vi "FPGA Toplevel.vi"() -> ()   [LabVIEW 2012]
uses:
  <vilib>/LabVIEW Targets/FPGA/RIO/BlueMoonOnboardIO/nicrio_cRIO-BlueMoonOnboardAi_TerminalMod.ctl
  <vilib>/LabVIEW Targets/FPGA/RIO/BlueMoonOnboardIO/nicrio_cRIO-BlueMoonOnboardAi_VoltageRange.ctl
  <vilib>/IEDriver/SPIandI2C/FPGA/Private/Initialize Port (I2C).vi
  <vilib>/IEDriver/SPIandI2C/FPGA/Private/IP Port (I2C).vi
  <vilib>/IEDriver/SPIandI2C/FPGA/Private/Configure Port (I2C).vi
  <vilib>/IEDriver/SPIandI2C/FPGA/Private/Read Port (I2C).vi
  <vilib>/IEDriver/SPIandI2C/FPGA/Private/Arm Port (I2C).vi
  <vilib>/IEDriver/SPIandI2C/FPGA/Private/Write Port (I2C).vi
  <vilib>/rvi/Emulation/niFpgaSctlEmulationGetInTimedLoop.vi
  <vilib>/rvi/Emulation/niFpgaSctlEmulationGlobalWrite.vi
  <vilib>/robotics/Utilities/FPGA Utilities/Generate Digital Pulse (uSec).vi
  <vilib>/rvi/eio/common/nirviEmuTemplateMethod_errors.vi
  <vilib>/rvi/eio/common/nirviEmuTemplatePropertySet_noerrors.vi
  <vilib>/eio/EIONode/EIONode.xnode
  <vilib>/eio/EIOPropertyNode/EIOPropertyNode.xnode
  <vilib>/rvi/eio/common/nirviEmuTemplatePropertyGet_errors.vi
  <vilib>/rvi/eio/common/nirviEmuTemplatePropertyGet_noerrors.vi
  <vilib>/rvi/eio/common/nirviEmuTemplatePropertySet_errors.vi
  <vilib>/robotics/Utilities/FPGA Utilities/NI_Robotics_FPGA Utilities.lvlib
  <vilib>/IEDriver/SPIandI2C/FPGA/Library/IP SPI&I2C.lvlib
panel:
  in  "servo Claw":u32=1500
  in  "Count(uSec) Claw":u32=5000
  in  "servo Arm":u32=1500
  in  "Count(uSec) Arm":u32=5000
  in  "Sensor time(us)":u16=1000 caption="Count(uSec)"
  in  "Calibration Parameters":T1={"m"=3.028200149536133, "b"=0.30049991607666016, "k"=0.04309988021850586}
  in  "Write Address":u8
  in  "Write Data In":u8
  out "Read Data out":u8
  in  "Read Address":u8
  in  "Mouse Action":T2(ring)
  out "IR 5":fxp<+/-,24,5>
  out "IR 4":fxp<+/-,24,5>
  out "IR 3":fxp<+/-,24,5>
  out "IR 2":fxp<+/-,24,5>
  in  "I2C Protocol Action 0":T3(ring)=enum."Idle"
  in  "I2C Protocol Input Data 0":u8
  out "I2C Protocol Output Data 0":u8
  in  "I2C Protocol Configure 0":T4 {"Command (Write & Read)" items=["Write & Read", "Write", "Read"]}
  out "IR 1":fxp<+/-,24,5>
  in  "Motor 4":T5={"Period (us)"=5000, "Pulse width (us)"=2502}
  in  "Motor 3":T5={"Period (us)"=5000, "Pulse width (us)"=2502}
  in  "Motor 2":T5={"Period (us)"=5000, "Pulse width (us)"=2502}
  in  "Enable":bool
  in  "Motor 1":refnum<k21>="DIO5"
  in  "Motor 1":T5={"Period (us)"=5000, "Pulse width (us)"=2502}
  in  "Enable":refnum<k21>="DIO4"
  in  "Motor 4":refnum<k21>="DIO8"
  in  "Motor 3":refnum<k21>="DIO7"
  in  "Motor 2":refnum<k21>="DIO6"
  out "IR 0":fxp<+/-,24,5>
  # "Mouse"
  # "Servo"
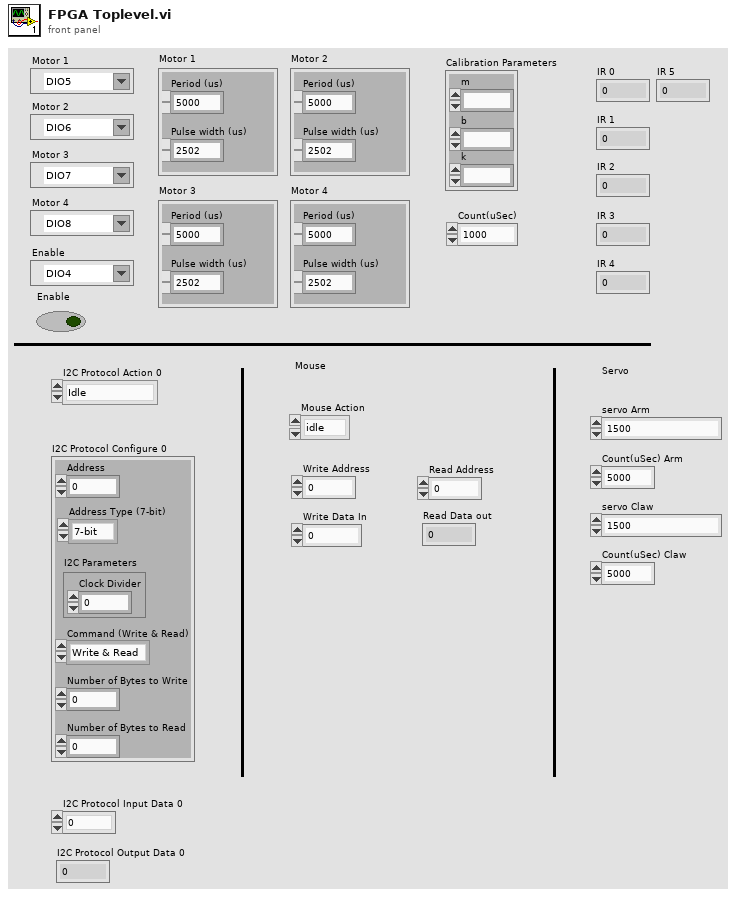
[diagram p1: front panel]
types:
  T1 = cluster{"m":fxp<+/-,26,5>, "b":fxp<+/-,26,5>, "k":fxp<+/-,26,5>}
  T2 = enum16{"idle", "set idle", "begin", "write", "read", "power down", "reset"}
  T3 = enum8{"Configure", "Write", "Arm", "Read", "Set Idle", "Idle"}
  T4 = cluster{"Address":u16, "Address Type (7-bit)":enum16{"7-bit", "10-bit"}, "I2C Parameters":cluster{"Clock Divider":u32}, "Command (Write & Read)":u8, "Number of Bytes to Write":u16, "Number of Bytes to Read":u16}
  T5 = cluster{"Period (us)":u32, "Pulse width (us)":u32}
  T6 = cluster{"SCL":refnum<k21>, "SDA":refnum<k21>, "PD":refnum<k21>}
  T7 = typedef "nicrio_cRIO-BlueMoonOnboardAi_TerminalMod.ctl" = u8
  T8 = typedef "nicrio_cRIO-BlueMoonOnboardAi_VoltageRange.ctl" = u8
  T9 = typedef "IP SPI&I2C.lvlib/Private Data (I2C).ctl" = cluster{"Arm Trigger":refnum<k21>, "API to IP Data":refnum<k21>, "IP to API Data":refnum<k21>, "Configuration Register":refnum<k21>, "Configuration Lock":refnum<k21>}
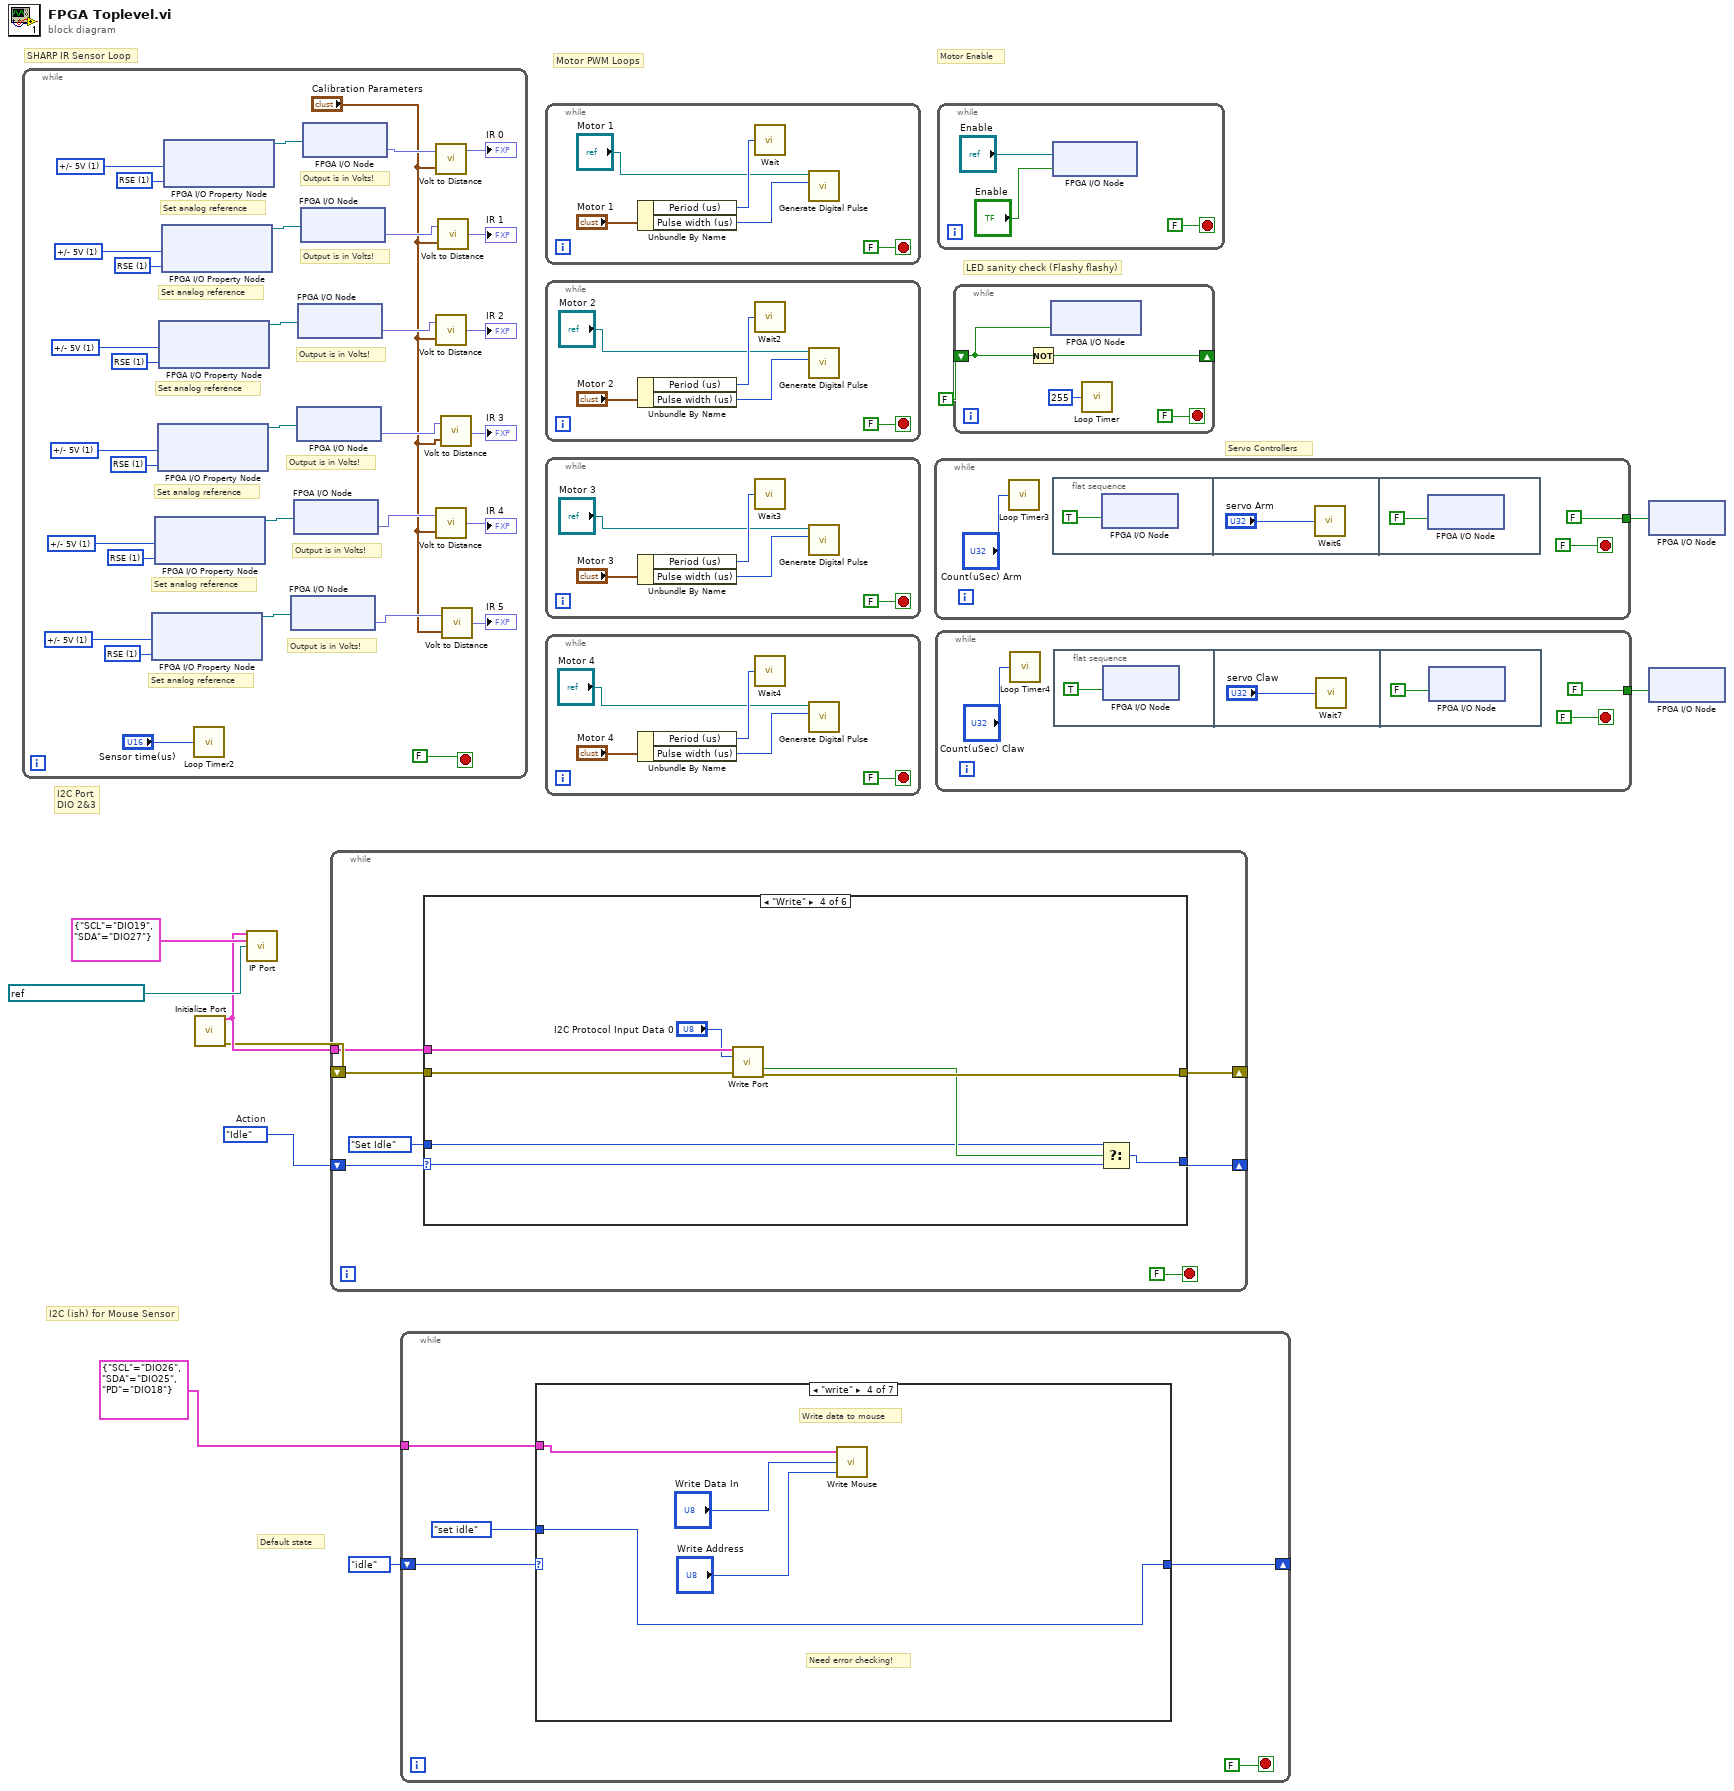
[diagram p0: block diagram]
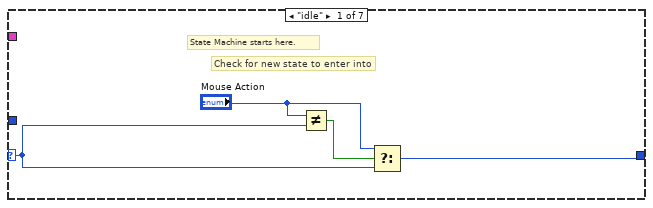
[diagram p2: hidden frame]
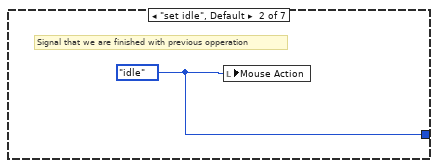
[diagram p3: hidden frame]
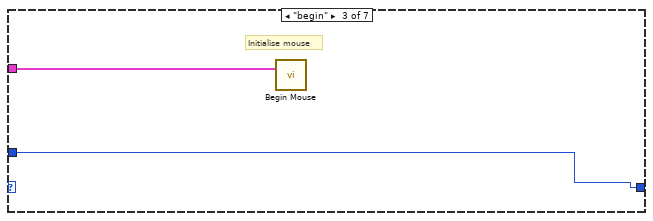
[diagram p4: hidden frame]
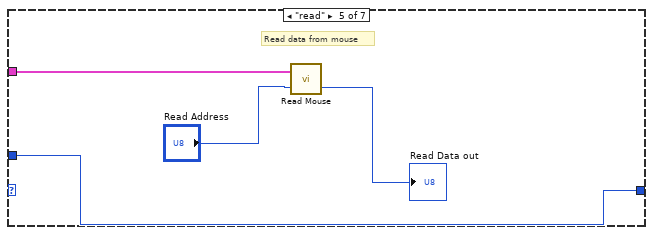
[diagram p5: hidden frame]
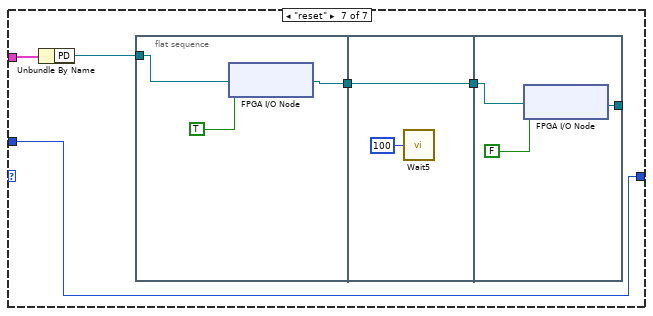
[diagram p7: hidden frame]
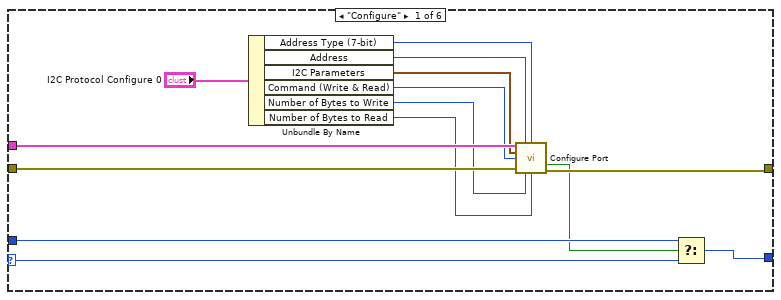
[diagram p8: hidden frame]
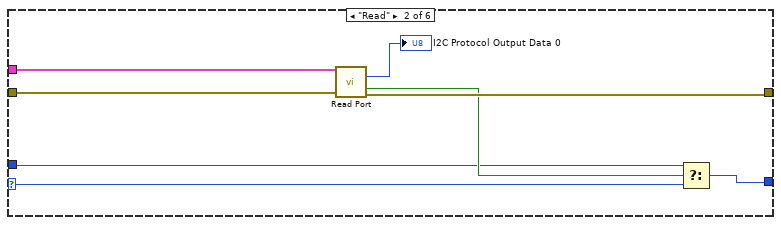
[diagram p9: hidden frame]
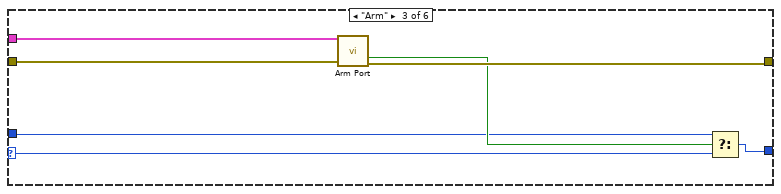
[diagram p10: hidden frame]
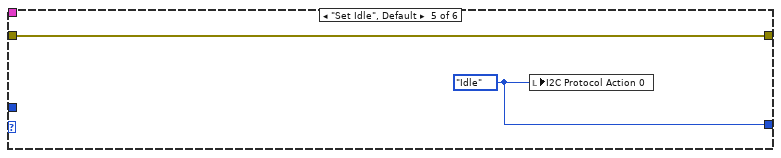
[diagram p11: hidden frame]
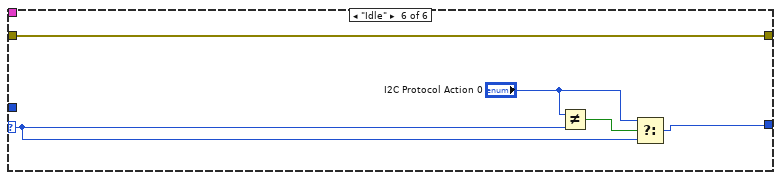
[diagram p12: hidden frame]
diagram:
  w6 = T3."Idle"  # Action
  # "Servo Controllers"
  # "LED sanity check (Flashy flashy)"
  # "Default state"
  # "I2C (ish) for Mouse Sensor"
  # "I2C Port\nDIO 2&3"
  # "Motor PWM Loops"
  # "Motor Enable"
  # "SHARP IR Sensor Loop"
  n1 = while {
    stop <- FALSE stop-if-true
    w27 = T7 1 items=["DIFF", "RSE"] ("Terminal Mode")
    w26 = T8 1 items=["+/- 10V", "+/- 5V", "+/- 2V", "+/- 1V"] ("Voltage Range")
    w28 = T7 1 items=["DIFF", "RSE"] ("Terminal Mode")
    w29 = T8 1 items=["+/- 10V", "+/- 5V", "+/- 2V", "+/- 1V"] ("Voltage Range")
    w33 = T7 1 items=["DIFF", "RSE"] ("Terminal Mode")
    w32 = T8 1 items=["+/- 10V", "+/- 5V", "+/- 2V", "+/- 1V"] ("Voltage Range")
    w34 = T7 1 items=["DIFF", "RSE"] ("Terminal Mode")
    w35 = T8 1 items=["+/- 10V", "+/- 5V", "+/- 2V", "+/- 1V"] ("Voltage Range")
    w39 = T7 1 items=["DIFF", "RSE"] ("Terminal Mode")
    w38 = T8 1 items=["+/- 10V", "+/- 5V", "+/- 2V", "+/- 1V"] ("Voltage Range")
    w40 = T7 1 items=["DIFF", "RSE"] ("Terminal Mode")
    w41 = T8 1 items=["+/- 10V", "+/- 5V", "+/- 2V", "+/- 1V"] ("Voltage Range")
    # "Output is in Volts!"
    # "Set analog reference"
    # "Output is in Volts!"
    # "Set analog reference"
    # "Output is in Volts!"
    # "Set analog reference"
    # "Output is in Volts!"
    # "Set analog reference"
    # "Output is in Volts!"
    # "Set analog reference"
    # "Output is in Volts!"
    # "Set analog reference"
    n2 = xnode "FPGA I/O Property Node"("Voltage Range"=w26, "Terminal Mode"=w27) -> ("FPGA I/O Out"=w25:refnum<k21>)  [unwired: 1 in]
    n3 = xnode "FPGA I/O Property Node"("Voltage Range"=w29, "Terminal Mode"=w28) -> ("FPGA I/O Out"=w30:refnum<k21>)  [unwired: 1 in]
    n4 = xnode "FPGA I/O Property Node"("Voltage Range"=w32, "Terminal Mode"=w33) -> ("FPGA I/O Out"=w31:refnum<k21>)  [unwired: 1 in]
    n5 = xnode "FPGA I/O Property Node"("Voltage Range"=w35, "Terminal Mode"=w34) -> ("FPGA I/O Out"=w36:refnum<k21>)  [unwired: 1 in]
    n6 = xnode "FPGA I/O Property Node"("Voltage Range"=w38, "Terminal Mode"=w39) -> ("FPGA I/O Out"=w37:refnum<k21>)  [unwired: 1 in]
    n7 = xnode "FPGA I/O Property Node"("Voltage Range"=w41, "Terminal Mode"=w40) -> ("FPGA I/O Out"=w42:refnum<k21>)  [unwired: 1 in]
    n8 = call "Loop Timer2"("Count(uSec)"="Sensor time(us)") -> ()  [unwired: 1 out]
    n9 = xnode "FPGA I/O Node"("FPGA I/O In"=w25) -> ("I/O Item"=w16:fxp<+/-,24,5>)  [unwired: 1 out]
    n10 = xnode "FPGA I/O Node"("FPGA I/O In"=w30) -> ("I/O Item"=w17:fxp<+/-,24,5>)  [unwired: 1 out]
    n11 = xnode "FPGA I/O Node"("FPGA I/O In"=w31) -> ("I/O Item"=w18:fxp<+/-,24,5>)  [unwired: 1 out]
    n12 = xnode "FPGA I/O Node"("FPGA I/O In"=w36) -> ("I/O Item"=w15:fxp<+/-,24,5>)  [unwired: 1 out]
    n13 = xnode "FPGA I/O Node"("FPGA I/O In"=w37) -> ("I/O Item"=w14:fxp<+/-,24,5>)  [unwired: 1 out]
    n14 = xnode "FPGA I/O Node"("FPGA I/O In"=w42) -> ("I/O Item"=w24:fxp<+/-,24,5>)  [unwired: 1 out]
    n15 = call "Volt to Distance.vi"("Calibration Parameters"="Calibration Parameters", "Voltage"=w24) -> ("Distance"=→"IR 0":fxp<+/-,26,5>)
    n16 = call "Volt to Distance.vi"("Calibration Parameters"="Calibration Parameters", "Voltage"=w15) -> ("Distance"=→"IR 2":fxp<+/-,26,5>)
    n17 = call "Volt to Distance.vi"("Calibration Parameters"="Calibration Parameters", "Voltage"=w17) -> ("Distance"=→"IR 4":fxp<+/-,26,5>)
    n18 = call "Volt to Distance.vi"("Calibration Parameters"="Calibration Parameters", "Voltage"=w14) -> ("Distance"=→"IR 1":fxp<+/-,26,5>)
    n19 = call "Volt to Distance.vi"("Calibration Parameters"="Calibration Parameters", "Voltage"=w18) -> ("Distance"=→"IR 3":fxp<+/-,26,5>)
    n20 = call "Volt to Distance.vi"("Calibration Parameters"="Calibration Parameters", "Voltage"=w16) -> ("Distance"=→"IR 5":fxp<+/-,26,5>)
  }
  n21 = call-poly <vilib>:"Initialize Port.vi"() -> ("Private Data Out"=w8:T9, "error out"=w7:errorcluster)  [unwired: 14 in]
  n22 = call-poly <vilib>:"IP Port.vi"("Private Data In"=w8, "I2C FPGA IO"=cluster{"SCL":refnum<k21>, "SDA":refnum<k21>} {"SCL"="DIO19", "SDA"="DIO27"}, "FPGA Clock"=refnum<k21> "40 MHz Onboard Clock") -> ()  [unwired: 13 in]
  n23 = while {
    shift-right: [w47] -> _
    shift-left: w7 -> [w49]
    tunnel: w8 -> [w50]
    shift-right: [w45] -> _
    shift-left: w6 -> [w46]
    stop <- FALSE stop-if-true
    n24 = case shown="\"Write\"" w46 {
      selector: w46 -> [w55 w66 w74 w81 _ w91]
      tunnel: w50 -> [w64 w72 w79 w87 _ _]
      tunnel: w49 -> [w63 w71 w78 w86 w89 w94]
      tunnel: [w62 w70 w77 w85 w89 w94] -> w47
      tunnel: [w56 w68 w76 w82 w88 w90] -> w45
      tunnel: T3."Set Idle" ("Action") -> [w54 w65 w73 w80 _ _]
      frame "Configure" {
        n25 = Unbundle By Name("I2C Protocol Configure 0") -> ("Address Type (7-bit)"=w60:enum16{"7-bit", "10-bit"}, "Address"=w51:u16, "I2C Parameters"=w59:cluster{"Clock Divider":u32}, "Command (Write & Read)"=w52:u8, "Number of Bytes to Write"=w58:u16, "Number of Bytes to Read"=w57:u16)
        n26 = call-poly <vilib>:"Configure Port.vi"("Private Data In"=w64, "Address"=w51, "Address Type (7-bit)"=w60, "I2C Parameters"=w59, "Command (Write & Read)"=w52, "error in"=w63, "Number of Bytes to Write"=w58, "Number of Bytes to Read"=w57) -> ("Done"=w53:bool, "error out"=w62:errorcluster)  [unwired: 5 in, 1 out]
        n27 = Select(t=w54, s=w53, f=w55) -> (s? t:f=w56:T3)
      }
      frame "Read" {
        n28 = call-poly <vilib>:"Read Port.vi"("Private Data In"=w72, "error in"=w71) -> ("Data Out"=→"I2C Protocol Output Data 0":u8, "Output Valid"=w67:bool, "error out"=w70:errorcluster)  [unwired: 10 in, 1 out]
        n29 = Select(t=w65, s=w67, f=w66) -> (s? t:f=w68:T3)
      }
      frame "Arm" {
        n30 = call-poly <vilib>:"Arm Port.vi"("Private Data In"=w79, "error in"=w78) -> ("Done"=w75:bool, "error out"=w77:errorcluster)  [unwired: 11 in, 1 out]
        n31 = Select(t=w73, s=w75, f=w74) -> (s? t:f=w76:T3)
      }
      frame "Write" {
        n32 = call-poly <vilib>:"Write Port.vi"("Private Data In"=w87, "Data In"="I2C Protocol Input Data 0", "error in"=w86) -> ("Done"=w83:bool, "error out"=w85:errorcluster)  [unwired: 10 in, 1 out]
        n33 = Select(t=w80, s=w83, f=w81) -> (s? t:f=w82:T3)
      }
      frame "Set Idle", Default {
        w88 = T3."Idle" ("Action")
        n34 = local write "I2C Protocol Action 0"(w88) -> ()
      }
      frame "Idle" {
        n35 = Not Equal?(x="I2C Protocol Action 0", y=w91) -> (x != y?=w93:bool)
        n36 = Select(t="I2C Protocol Action 0", s=w93, f=w91) -> (s? t:f=w90:T3)
      }
    }
  }
  n37 = while {
    tunnel: T6 {"SCL"="DIO26", "SDA"="DIO25", "PD"="DIO18"} ("Mouse IO") -> [w98]
    shift-right: [w97] -> _
    shift-left: T2."idle" ("Mouse Action") -> [w96]
    stop <- FALSE stop-if-true
    n38 = case shown="\"write\"" w96 {
      selector: w96 -> [w102 _ _ _ _ _ _]
      tunnel: w98 -> [_ _ w106 w109 w114 _ w120]
      tunnel: [w101 w104 w105 w110 w111 w115 w116] -> w97
      tunnel: T2."set idle" ("Mouse Action") -> [_ _ w105 w110 w111 w115 w116]
      frame "idle" {
        # "Check for new state to enter into"
        # "State Machine starts here."
        n39 = Not Equal?(x="Mouse Action", y=w102) -> (x != y?=w103:bool)
        n40 = Select(t="Mouse Action", s=w103, f=w102) -> (s? t:f=w101:T2)
      }
      frame "set idle", Default {
        w104 = T2."idle" ("Mouse Action")
        # "Signal that we are finished with previous opperation"
        n41 = local write "Mouse Action"(w104) -> ()
      }
      frame "begin" {
        # "Initialise mouse"
        n42 = call "Begin Mouse.vi"("Mouse IO"=w106) -> ()  [unwired: 2 in, 1 out]
      }
      frame "write" {
        # "Need error checking!"
        # "Write data to mouse"
        n43 = call "Write Mouse.vi"("Write Address"="Write Address", "Data In"="Write Data In", "Mouse IO"=w109) -> ()  [unwired: 2 in, 1 out]
      }
      frame "read" {
        # "Read data from mouse"
        n44 = call "Read Mouse.vi"("Read Address"="Read Address", "Mouse IO"=w114) -> ("Data out"=→"Read Data out":u8)  [unwired: 1 out]
      }
      frame "power down" {
      }
      frame "reset" {
        n45 = Unbundle By Name(w120) -> ("PD"=w119:refnum<k21>)
        n46 = flat-sequence {
          tunnel: w119 -> [w123]
          tunnel: [w122] -> w118
          tunnel: w118 -> [w124]
          tunnel: [w124] -> w117
          tunnel: w117 -> [w127]
          tunnel: [w126] -> _
          frame #0 {
            n47 = xnode "FPGA I/O Node"("I/O Item"=TRUE, "FPGA I/O In"=w123) -> ("FPGA I/O Out"=w122:refnum<k21>)
          }
          frame #1 {
            n48 = call "Wait5"("Count(uSec)"=u8 100) -> ()  [unwired: 1 out]
          }
          frame #2 {
            n49 = xnode "FPGA I/O Node"("I/O Item"=FALSE, "FPGA I/O In"=w127) -> ("FPGA I/O Out"=w126:refnum<k21>)
          }
        }
      }
    }
  }
  n50 = while {
    stop <- FALSE stop-if-true
    n51 = Unbundle By Name("Motor 1") -> ("Period (us)"=w131:u32, "Pulse width (us)"=w132:u32)
    n52 = call "Wait"("Count(uSec)"=w131) -> ()  [unwired: 1 out]
    n53 = call-poly <vilib>:"Generate Digital Pulse.vi"("pulse width (uSec)"=w132, "FPGA digital output"="Motor 1") -> ()  [unwired: 10 in]
  }
  n54 = while {
    stop <- FALSE stop-if-true
    n55 = Unbundle By Name("Motor 2") -> ("Period (us)"=w136:u32, "Pulse width (us)"=w137:u32)
    n56 = call "Wait2"("Count(uSec)"=w136) -> ()  [unwired: 1 out]
    n57 = call-poly <vilib>:"Generate Digital Pulse.vi"("pulse width (uSec)"=w137, "FPGA digital output"="Motor 2") -> ()  [unwired: 10 in]
  }
  n58 = while {
    stop <- FALSE stop-if-true
    n59 = Unbundle By Name("Motor 3") -> ("Period (us)"=w141:u32, "Pulse width (us)"=w142:u32)
    n60 = call "Wait3"("Count(uSec)"=w141) -> ()  [unwired: 1 out]
    n61 = call-poly <vilib>:"Generate Digital Pulse.vi"("pulse width (uSec)"=w142, "FPGA digital output"="Motor 3") -> ()  [unwired: 10 in]
  }
  n62 = while {
    stop <- FALSE stop-if-true
    n63 = Unbundle By Name("Motor 4") -> ("Period (us)"=w146:u32, "Pulse width (us)"=w147:u32)
    n64 = call "Wait4"("Count(uSec)"=w146) -> ()  [unwired: 1 out]
    n65 = call-poly <vilib>:"Generate Digital Pulse.vi"("pulse width (uSec)"=w147, "FPGA digital output"="Motor 4") -> ()  [unwired: 10 in]
  }
  n66 = while {
    tunnel: [FALSE ("Mod1/DO0")] -> w2
    stop <- FALSE stop-if-true
    n67 = call "Loop Timer3"("Count(uSec)"="Count(uSec) Arm") -> ()  [unwired: 1 out]
    n68 = flat-sequence {
      frame #0 {
        n69 = xnode "FPGA I/O Node"("DIO0"=TRUE) -> ()  [unwired: 1 in, 1 out]
      }
      frame #1 {
        n70 = call "Wait6"("Count(uSec)"="servo Arm") -> ()  [unwired: 1 out]
      }
      frame #2 {
        n71 = xnode "FPGA I/O Node"("DIO0"=FALSE) -> ()  [unwired: 1 in, 1 out]
      }
    }
  }
  n72 = while {
    tunnel: [FALSE ("Mod1/DO0")] -> w1
    stop <- FALSE stop-if-true
    n73 = call "Loop Timer4"("Count(uSec)"="Count(uSec) Claw") -> ()  [unwired: 1 out]
    n74 = flat-sequence {
      frame #0 {
        n75 = xnode "FPGA I/O Node"("DIO1"=TRUE) -> ()  [unwired: 1 in, 1 out]
      }
      frame #1 {
        n76 = call "Wait7"("Count(uSec)"="servo Claw") -> ()  [unwired: 1 out]
      }
      frame #2 {
        n77 = xnode "FPGA I/O Node"("DIO1"=FALSE) -> ()  [unwired: 1 in, 1 out]
      }
    }
  }
  n78 = while {
    stop <- FALSE stop-if-true
    n79 = xnode "FPGA I/O Node"("I/O Item"="Enable", "FPGA I/O In"="Enable") -> ()  [unwired: 1 out]
  }
  n80 = while {
    shift-right: [w165] -> _
    shift-left: FALSE -> [w166]
    stop <- FALSE stop-if-true
    n81 = Not(x=w166) -> (.not. x?=w165:bool)
    n82 = xnode "FPGA I/O Node"("FPGA LED"=w166) -> ()  [unwired: 1 in, 1 out]
    n83 = call "Loop Timer"("Count(mSec)"=u8 255) -> ()  [unwired: 1 out]
  }
  n84 = xnode "FPGA I/O Node"("DIO0"=w2) -> ()  [unwired: 1 in, 1 out]
  n85 = xnode "FPGA I/O Node"("DIO1"=w1) -> ()  [unwired: 1 in, 1 out]
